vi "FTW-Test-Actor-Core_Process.vi"(0 "FTW Actor Instance Configuration":string="{\n  \"Identity\": \"ActorName\",\n  \"InboxAddress\": \"inproc://*\",\n  \"LoggerAddress\": \"\",\n  \"My Data\": false,\n  \"Publisher URI\": \"inproc://*\",\n  \"Subscriber URIs\": \"\",\n  \"Refresh Period\": 2\n}", 11 "ErrorIn":errorcluster) -> (15 "Error":errorcluster)   [LabVIEW 2015, in "FTW-Test-Actor-Core.lvclass"]
uses:
  FTW-Test-Actor-Core.lvclass
  source/actor/Message/Base/FTW-Message.lvclass
  FTW-Test-Actor-Core.lvclass/FTW-Test-Actor-Core.ctl
  source/actor/Instance/FTW-ActorInstance.lvclass/FTW-ActorInstance.ctl
  source/actor/JobSequencer/FTW-SEQ-Current.vi
  source/actor/Connector/FTW-ActorConnector.lvclass
  source/actor/Instance/FTW-ActorInstance.lvclass
  source/actor/Message/Request/FTW-Message-IncomingRequest.lvclass
  source/actor/Publisher/FTW-Publisher.lvclass
  source/actor/Subscriber/FTW-Subscriber.lvclass
panel:
  # "#TODO\nhide controls for a GUI"
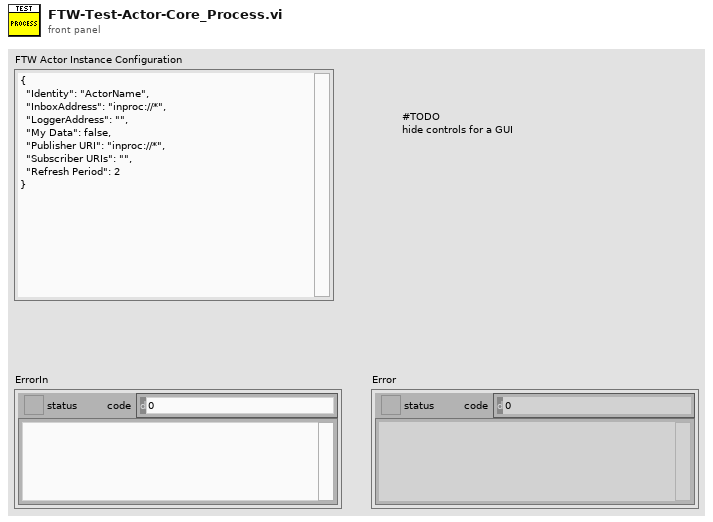
[diagram p1: front panel]
types:
  T1 = cluster{"Incoming Requests":refnum<event-registration>, "Local Messages":refnum<event-registration>, "Subscription":refnum<event-registration>}
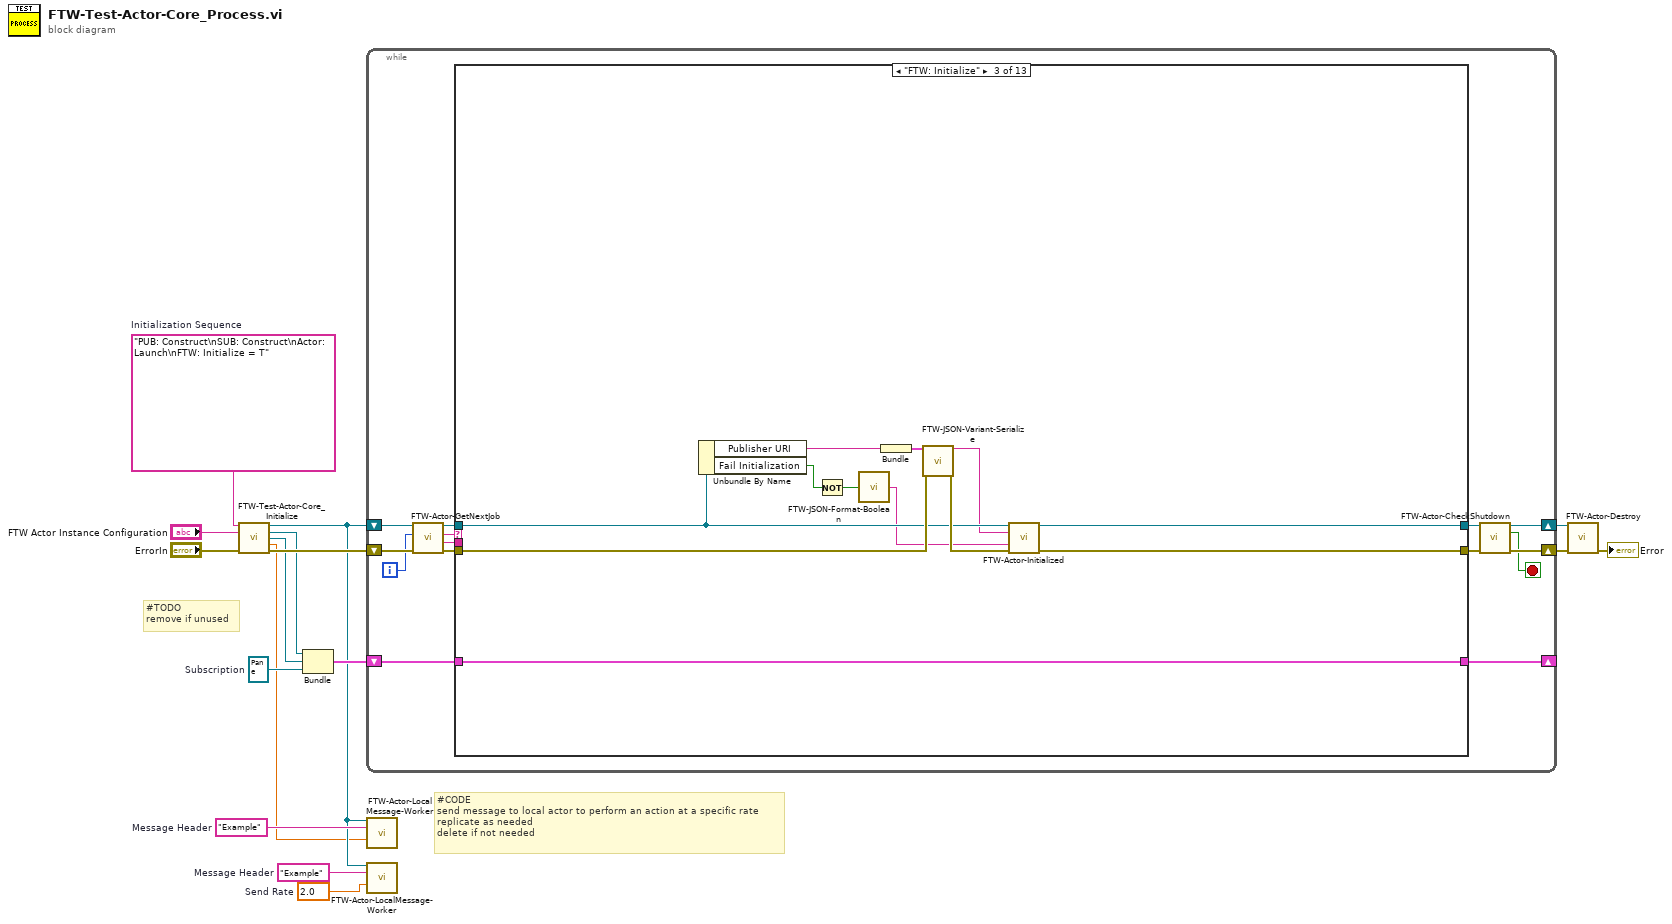
[diagram p0: block diagram]
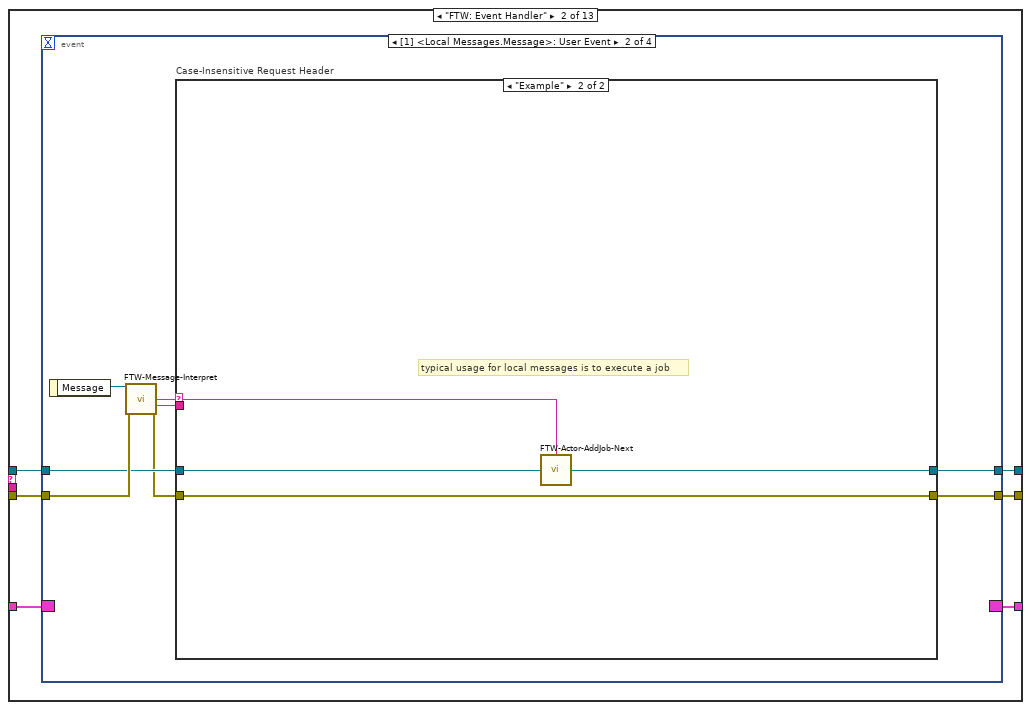
[diagram p3: hidden frame]
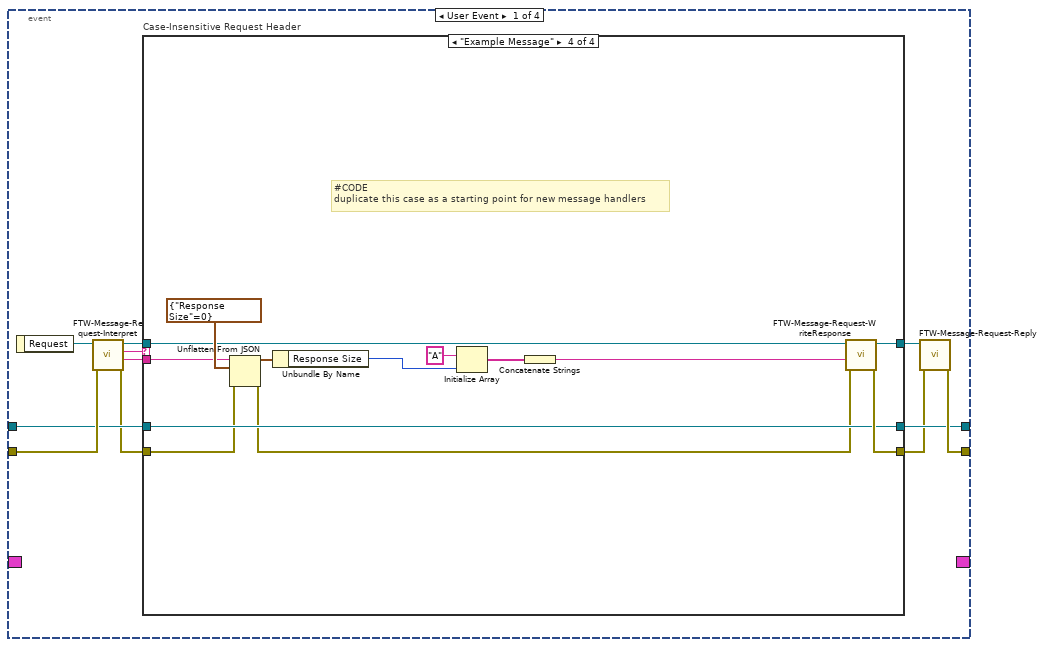
[diagram p4: hidden frame]
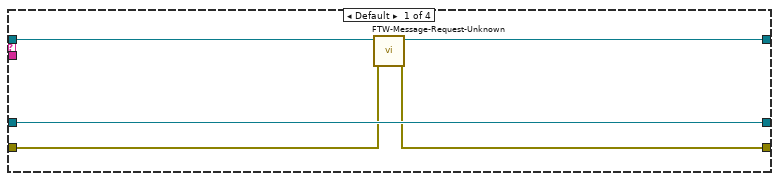
[diagram p5: hidden frame]
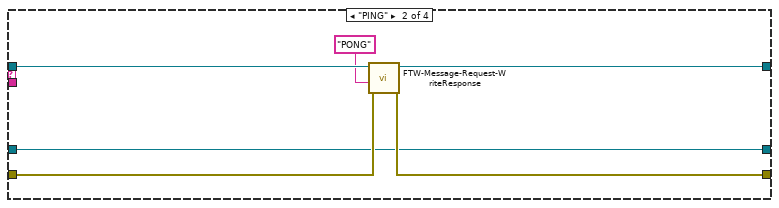
[diagram p6: hidden frame]
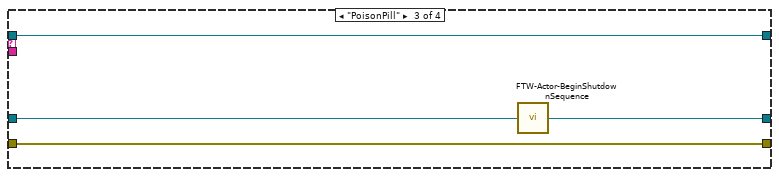
[diagram p7: hidden frame]
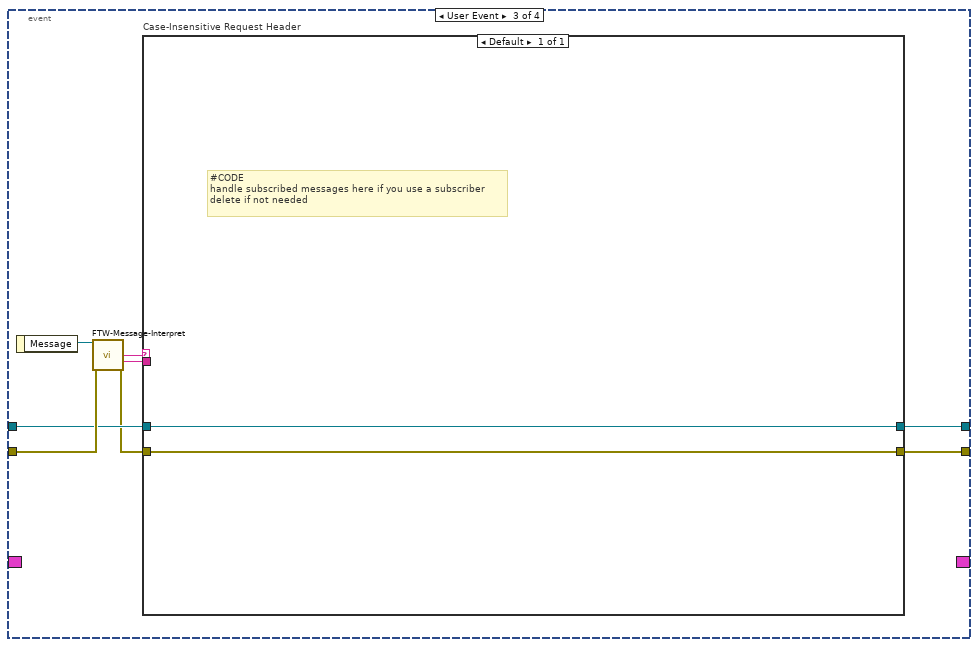
[diagram p9: hidden frame]
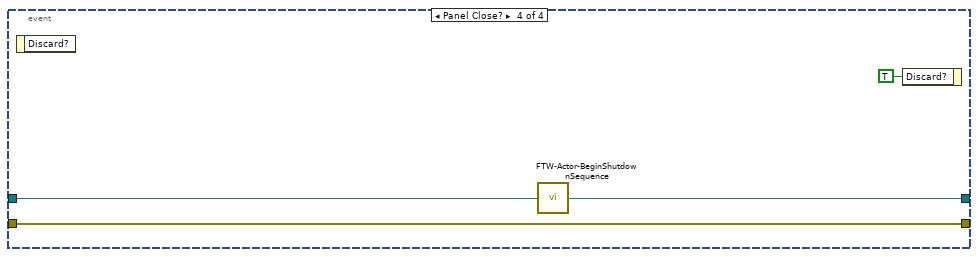
[diagram p10: hidden frame]
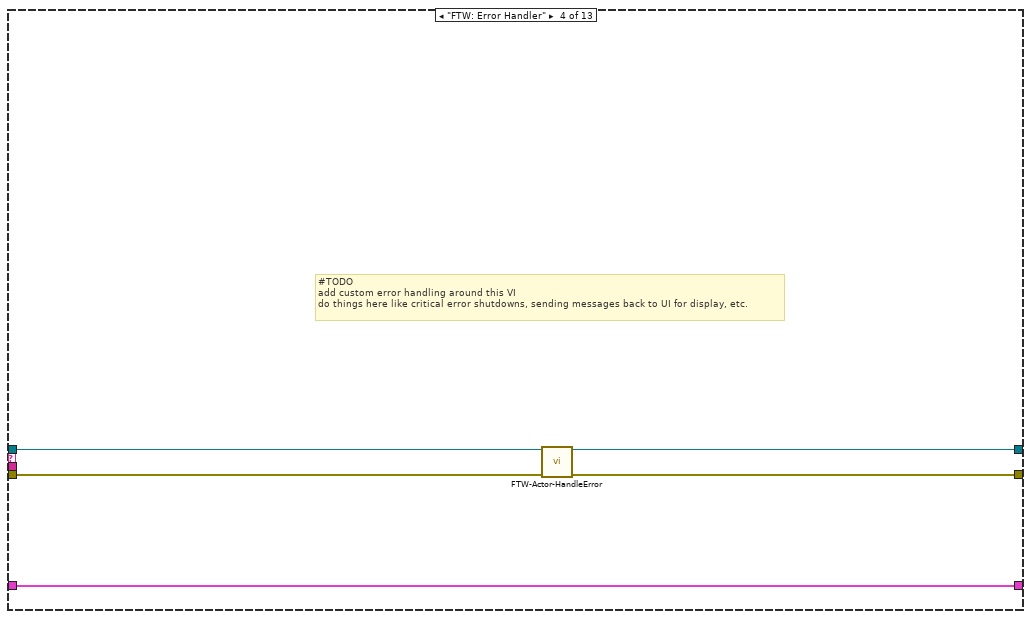
[diagram p11: hidden frame]
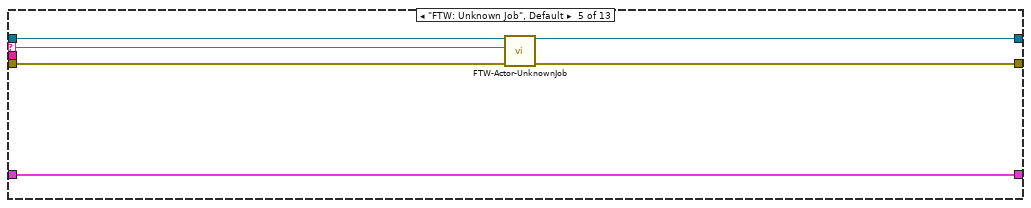
[diagram p12: hidden frame]
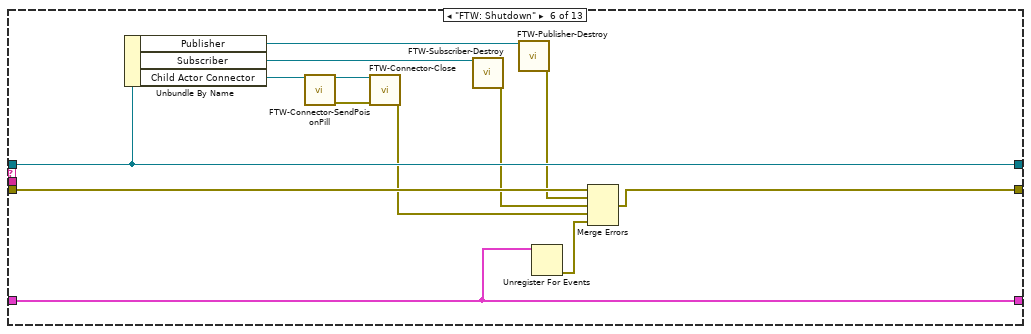
[diagram p13: hidden frame]
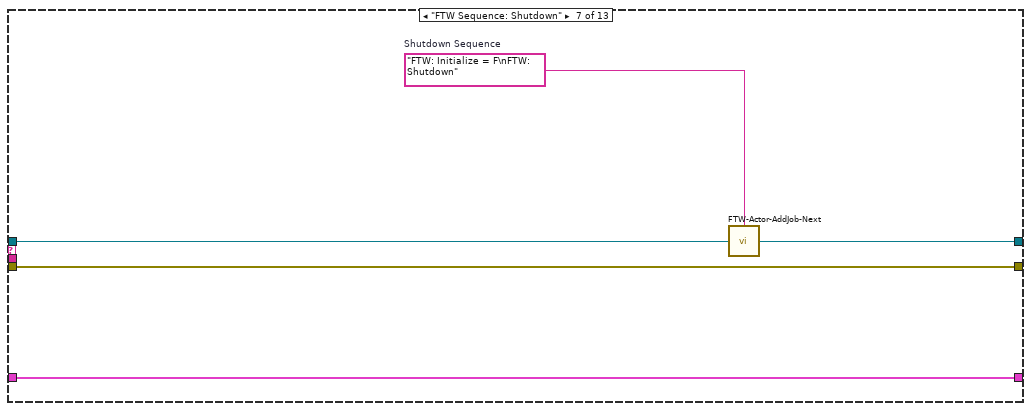
[diagram p14: hidden frame]
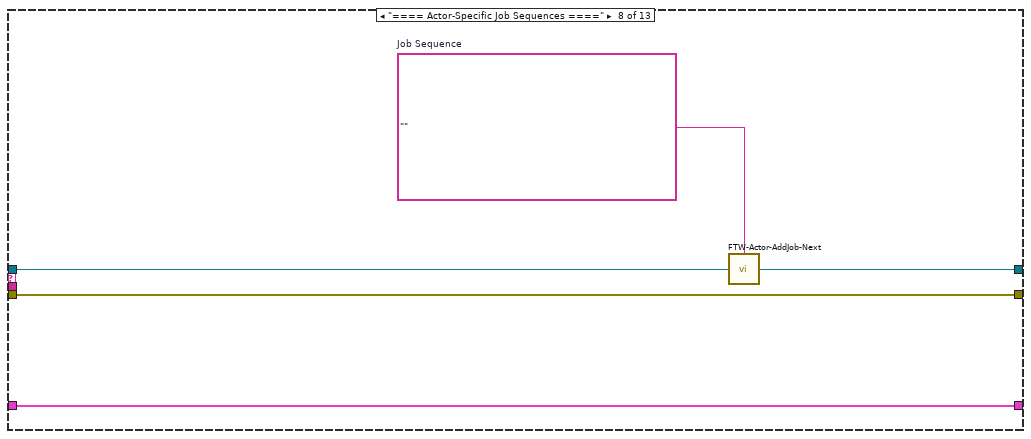
[diagram p15: hidden frame]
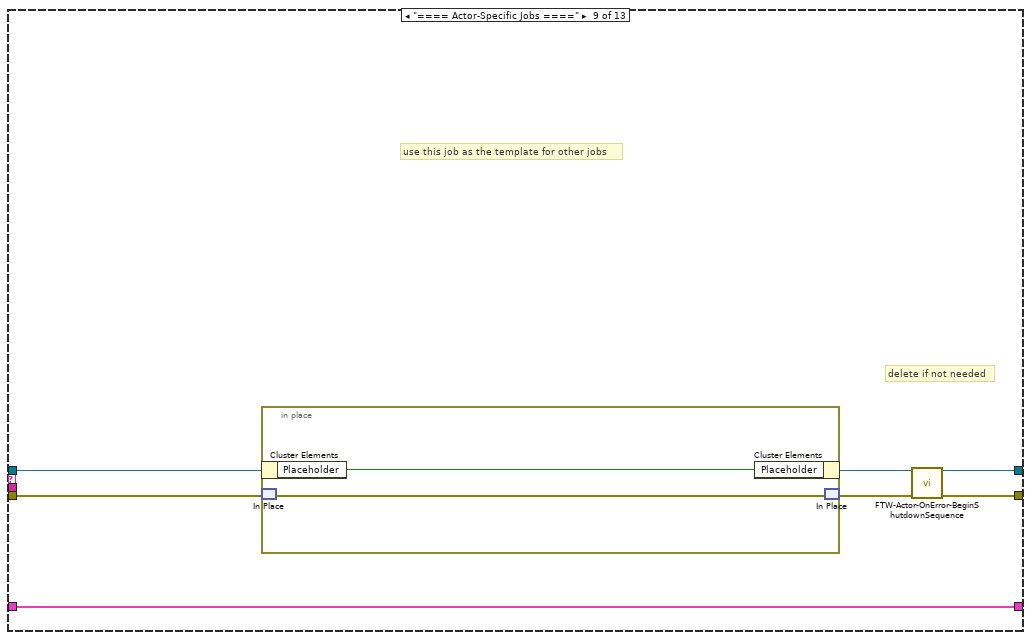
[diagram p16: hidden frame]
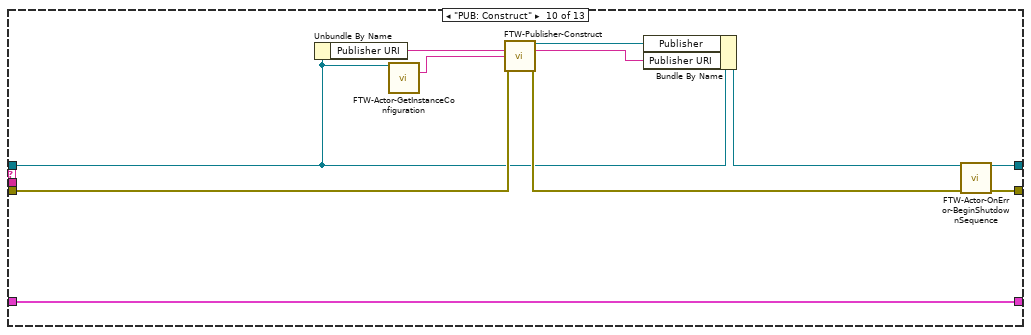
[diagram p17: hidden frame]
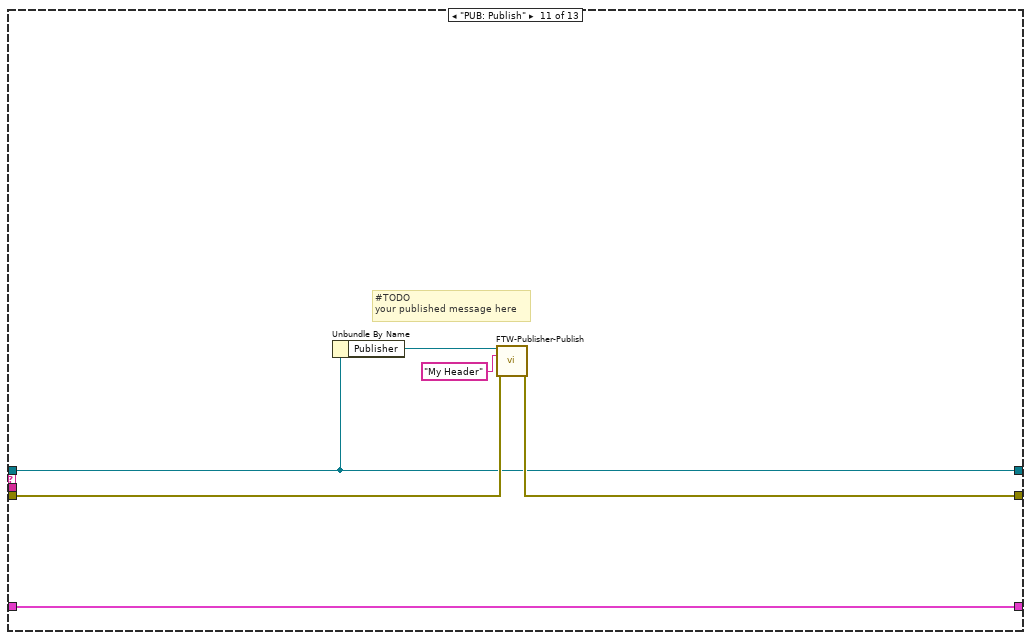
[diagram p18: hidden frame]
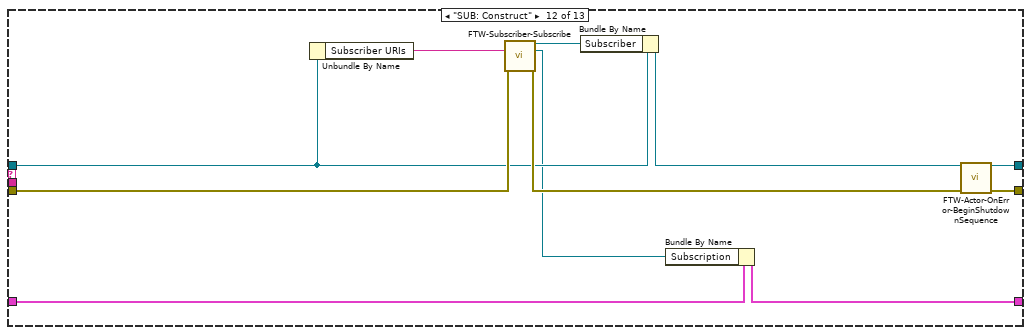
[diagram p19: hidden frame]
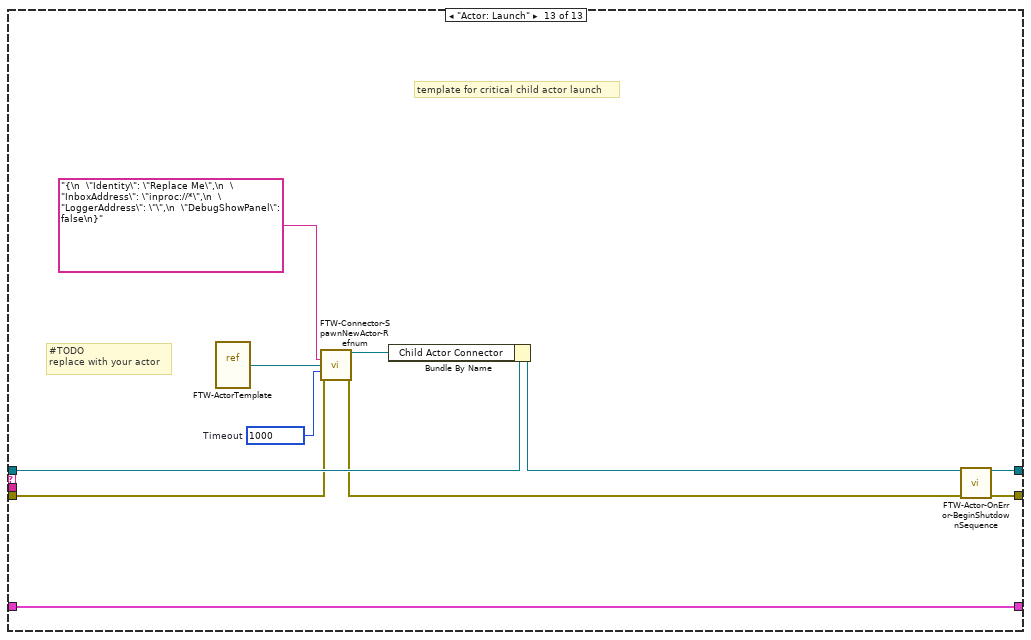
[diagram p20: hidden frame]
diagram:
  w4 = 2.0  # Send Rate
  w3 = "Example"  # Message Header
  w5 = "Example"  # Message Header
  w6 = refnum<event-registration> refnum  # Subscription
  w12 = "PUB: Construct\nSUB: Construct\nActor: Launch\nFTW: Initialize = T"  # Initialization Sequence
  # "#CODE\nsend message to local actor to perform an action at a specific rate\nreplicate as needed\ndelete if not needed"
  # "#TODO\nremove if unused"
  n1 = call "FTW-Test-Actor-Core_Initialize.vi"("Initialization Sequence"=w12, "FTW Actor Instance Configuration"="FTW Actor Instance Configuration", "error in (no error)"="ErrorIn") -> ("Actor Template-Core out"=w2:refnum<class "FTW-Test-Actor-Core.lvclass">, "Incoming Requests"=w8:refnum<event-registration>, "Local Messages"=w7:refnum<event-registration>, "Refresh Period"=w1:dbl, "error out"=w13:errorcluster)  [unwired: 8 in]
  n2 = Bundle("Incoming Requests"=w8, "Local Messages"=w7, "Subscription"=w6) -> (w10:T1)  [unwired: 1 in]
  n3 = while {
    shift-right: [w20] -> w15
    shift-left: w13 -> [w27]
    shift-right: [w17] -> _
    shift-left: w10 -> [w30]
    shift-right: [w22] -> w16
    shift-left: w2 -> [w29]
    i -> [w18]
    stop <- w19 stop-if-true
    n4 = call "FTW-Actor-GetNextJob.vi"("error in"=w27, "Jobs Performed"=w18, "FTW Actor Instance"=w29) -> ("error out"=w26:errorcluster, "Job Data"=w24:string, "Job Name"=w25:string, "FTW Actor Instance out"=w28:refnum<class "FTW-Test-Actor-Core.lvclass">)  [unwired: 5 in]
    n5 = case shown="\"FTW: Initialize\"" w25 {
      selector: w25 -> [_ _ _ _ w124 _ _ _ _ _ _ _ _]
      tunnel: [w32 w39 w114 w119 w127 w141 w146 w151 w155 w168 w176 w185 w199] -> w21
      tunnel: w26 -> [w32 w38 w118 w121 w128 w142 w146 w151 w158 w170 w177 w187 w193]
      tunnel: w30 -> [w33 w34 w116 w123 w129 w139 w147 w152 w159 w172 w178 w189 w200]
      tunnel: [w33 w37 w116 w123 w129 w139 w147 w152 w159 w172 w178 w180 w200] -> w17
      tunnel: w24 -> [_ _ _ _ _ _ _ _ _ _ _ _ _]
      tunnel: [w31 w36 w115 w120 w125 w138 w144 w149 w153 w166 w175 w183 w198] -> w23
      tunnel: w28 -> [w31 w35 w113 w122 w126 w138 w145 w150 w156 w163 w175 w181 w197]
      frame "==== Featherweight Framework Jobs ====" {
      }
      frame "FTW: Event Handler" {
        n6 = event shown="[1] <Local Messages.Message>: User Event" {
          selector: w34 -> [_ _ _ _]
          dyn-events: [_ _ _ _] -> w37
          timeout: _ -> [_ _ _ _]
          tunnel: [w49 w81 w95 w105] -> w39
          tunnel: w38 -> [w48 w85 w99 w105]
          tunnel: [w43 w82 w96 w103] -> w36
          tunnel: w35 -> [w47 w84 w98 w104]
          event User Event {
            n7 = event-data() -> ("Request"=w50:refnum<class "FTW-Message-IncomingRequest.lvclass">)  [unwired: 1 in]
            n8 = call "FTW-Message-Request-Interpret.vi"("error in"=w48, "FTW Incoming Request"=w50) -> ("error out"=w46:errorcluster, "Request Body"=w40:string, "Request Header"=w44:string, "FTW Incoming Request out"=w45:refnum<class "FTW-Message-IncomingRequest.lvclass">)  [unwired: 6 in]
            n9 = case "Case-Insensitive Request Header" shown="\"Example Message\"" w44 {
              tunnel: [w53 w59 w64 w78] -> w42
              tunnel: w46 -> [w54 w60 w64 w67]
              tunnel: [w55 w58 w65 w76] -> w43
              tunnel: w47 -> [w55 w58 w63 w76]
              tunnel: w45 -> [w52 w61 w62 w68]
              tunnel: [w51 w57 w62 w77] -> w41
              tunnel: w40 -> [_ _ _ w66]
              frame Default {
                n10 = call "FTW-Message-Request-Unknown.vi"("error in"=w54, "FTW Incoming Request"=w52) -> ("error out"=w53:errorcluster, "FTW Incoming Request Out"=w51:refnum<class "FTW-Message-IncomingRequest.lvclass">)  [unwired: 8 in]
              }
              frame "PING" {
                n11 = call "FTW-Message-Request-WriteResponse.vi"("error in"=w60, "Response Body"="PONG" ("Response Header"), "FTW Incoming Request"=w61) -> ("error out"=w59:errorcluster, "FTW Incoming Request out"=w57:refnum<class "FTW-Message-IncomingRequest.lvclass">)  [unwired: 7 in]
              }
              frame "PoisonPill" {
                n12 = call "FTW-Actor-BeginShutdownSequence.vi"("FTW Actor Instance"=w63) -> ("FTW Actor Instance out"=w65:refnum<class "FTW-Test-Actor-Core.lvclass">)  [unwired: 3 in]
              }
              frame "Example Message" {
                # "#CODE\nduplicate this case as a starting point for new message handlers"
                n13 = Unflatten From JSON(JSON string=w66, type and defaults=cluster{"Response Size":i32} {"Response Size"=0}, error in (no error)=w67) -> (value=w73:cluster{"Response Size":i32}, error out=w75:errorcluster)  [unwired: 4 in]
                n14 = Unbundle By Name(w73) -> ("Response Size"=w72:i32)
                n15 = Initialize Array("A", w72) -> (w70:string[])
                n16 = Concatenate Strings(w70) -> (w69:string)
                n17 = call "FTW-Message-Request-WriteResponse.vi"("error in"=w75, "Response Body"=w69, "FTW Incoming Request"=w68) -> ("error out"=w78:errorcluster, "FTW Incoming Request out"=w77:refnum<class "FTW-Message-IncomingRequest.lvclass">)  [unwired: 7 in]
              }
            }
            n18 = call "FTW-Message-Request-Reply.vi"("FTW: Reply Error"=w42, "FTW Incoming Request"=w41) -> ("error out"=w49:errorcluster)  [unwired: 8 in, 1 out]
          }
          event User Event {
            n19 = event-data() -> ("Message"=w86:refnum<class "FTW-Message.lvclass">)  [unwired: 1 in]
            n20 = call-dynamic "FTW-Message-Interpret.vi"("FTW Message"=w86, "error in"=w85) -> ("Message Header"=w80:string, "Message Body"=w79:string, "error out"=w83:errorcluster)  [unwired: 9 in, 2 out]
            n21 = case "Case-Insensitive Request Header" shown="\"Example\"" w80 {
              selector: w80 -> [_ w89]
              tunnel: [w87 w91] -> w81
              tunnel: w83 -> [w87 w91]
              tunnel: [w88 w90] -> w82
              tunnel: w84 -> [w88 w92]
              tunnel: w79 -> [_ _]
              frame Default {
                # "#CODE\nhandle local messages here\ndelete if not needed"
              }
              frame "Example" {
                # "typical usage for local messages is to execute a job"
                n22 = call "FTW-Actor-AddJob-Next.vi"("Add Next in Job Queue"=w89, "FTW Actor Instance"=w92) -> ("FTW Actor Instance out"=w90:refnum<class "FTW-Test-Actor-Core.lvclass">)  [unwired: 2 in]
              }
            }
          }
          event User Event {
            n23 = event-data() -> ("Message"=w100:refnum<class "FTW-Message.lvclass">)  [unwired: 1 in]
            n24 = call-dynamic "FTW-Message-Interpret.vi"("FTW Message"=w100, "error in"=w99) -> ("Message Header"=w94:string, "Message Body"=w93:string, "error out"=w97:errorcluster)  [unwired: 9 in, 2 out]
            n25 = case "Case-Insensitive Request Header" shown="Default" w94 {
              tunnel: [w101] -> w95
              tunnel: w97 -> [w101]
              tunnel: [w102] -> w96
              tunnel: w98 -> [w102]
              tunnel: w93 -> [_]
              frame Default {
                # "#CODE\nhandle subscribed messages here if you use a subscriber\ndelete if not needed"
              }
            }
          }
          event Panel Close? {
            n26 = event-data() -> ()  [unwired: 1 in, 1 out]
            n27 = call "FTW-Actor-BeginShutdownSequence.vi"("FTW Actor Instance"=w104) -> ("FTW Actor Instance out"=w103:refnum<class "FTW-Test-Actor-Core.lvclass">)  [unwired: 3 in]
            n28 = event-data("Discard?"=TRUE) -> ()  [unwired: 1 in, 1 out]
          }
        }
      }
      frame "FTW: Initialize" {
        n29 = Unbundle By Name(w113) -> ("Publisher URI"=w112:string, "Fail Initialization"=w109:bool)
        n30 = Not(x=w109) -> (.not. x?=w107:bool)
        n31 = call "FTW-JSON-Format-Boolean.vi"("LabVIEW Boolean"=w107) -> ("JSON Boolean"=w108:string)
        n32 = Bundle("Publisher URI"=w112) -> (w111:cluster{"Publisher URI":string})  [unwired: 1 in]
        n33 = call "FTW-JSON-Variant-Serialize.vi"("Variant"=w111, "error in"=w118) -> ("JSON String"=w110:string, "error out"=w117:errorcluster)  [unwired: 12 in]
        n34 = call-dynamic "FTW-Actor-Initialized.vi"("FTW Actor Instance"=w113, "Initialized Response"=w110, "Positive Init?"=w108, "error in"=w117) -> ("FTW Actor Instance out"=w115:refnum<class "FTW-Test-Actor-Core.lvclass">, "error out"=w114:errorcluster)  [unwired: 10 in]
      }
      frame "FTW: Error Handler" {
        # "#TODO\nadd custom error handling around this VI\ndo things here like critical error shutdowns, sending messages back to UI for display, etc."
        n35 = call-dynamic "FTW-Actor-HandleError.vi"("FTW Actor Instance"=w122, "error in"=w121) -> ("FTW Actor Instance out"=w120:refnum<class "FTW-Test-Actor-Core.lvclass">, "error out"=w119:errorcluster)  [unwired: 10 in, 2 out]
      }
      frame "FTW: Unknown Job", Default {
        n36 = call-dynamic "FTW-Actor-UnknownJob.vi"("FTW Actor Instance"=w126, "Unknown Job"=w124, "error in"=w128) -> ("FTW Actor Instance out"=w125:refnum<class "FTW-Test-Actor-Core.lvclass">, "error out"=w127:errorcluster)  [unwired: 11 in]
      }
      frame "FTW: Shutdown" {
        n37 = Unbundle By Name(w138) -> ("Publisher"=w137:refnum<class "FTW-Publisher.lvclass">, "Subscriber"=w135:refnum<class "FTW-Subscriber.lvclass">, "Child Actor Connector"=w133:refnum<class "FTW-ActorConnector.lvclass">)
        n38 = call-dynamic "FTW-Connector-SendPoisonPill.vi"("FTW Actor Connector"=w133) -> ("FTW Actor Connector out"=w132:refnum<class "FTW-ActorConnector.lvclass">, "error out"=w131:errorcluster)  [unwired: 9 in, 4 out]
        n39 = call-dynamic "FTW-Connector-Close.vi"("FTW Actor Connector"=w132, "error in"=w131) -> ("error out"=w130:errorcluster)  [unwired: 13 in]
        n40 = call "FTW-Subscriber-Destroy.vi"("FTW-Subscription In"=w135) -> ("error out"=w134:errorcluster)  [unwired: 14 in]
        n41 = call "FTW-Publisher-Destroy.vi"("FTW-Publisher In"=w137) -> ("error out"=w136:errorcluster)  [unwired: 14 in]
        n42 = Unregister For Events(event registration refnum=w139) -> (error out=w140:errorcluster)  [unwired: 1 in]
        n43 = Merge Errors(w142, w136, w134, w130, w140) -> (w141:errorcluster)
      }
      frame "FTW Sequence: Shutdown" {
        w143 = "FTW: Initialize = F\nFTW: Shutdown"  # Shutdown Sequence
        n44 = call "FTW-Actor-AddJob-Next.vi"("Add Next in Job Queue"=w143, "FTW Actor Instance"=w145) -> ("FTW Actor Instance out"=w144:refnum<class "FTW-Test-Actor-Core.lvclass">)  [unwired: 2 in]
      }
      frame "==== Actor-Specific Job Sequences ====" {
        w148 = ""  # Job Sequence
        n45 = call "FTW-Actor-AddJob-Next.vi"("Add Next in Job Queue"=w148, "FTW Actor Instance"=w150) -> ("FTW Actor Instance out"=w149:refnum<class "FTW-Test-Actor-Core.lvclass">)  [unwired: 2 in]
      }
      frame "==== Actor-Specific Jobs ====" {
        # "delete if not needed"
        # "use this job as the template for other jobs"
        n46 = in-place {
          n47 = in-place-cluster #1(w156) -> ("Placeholder"=w160:bool)
          n48 = in-place-match #2(w158) -> (w161:errorcluster)
          n49 = in-place-cluster #1("Placeholder"=w160) -> (w154:refnum<class "FTW-Test-Actor-Core.lvclass">)
          n50 = in-place-match #2(w161) -> (w157:errorcluster)
        }
        n51 = call-dynamic "FTW-Actor-OnError-BeginShutdownSequence.vi"("FTW Actor Instance"=w154, "error in"=w157) -> ("FTW Actor Instance out"=w153:refnum<class "FTW-Test-Actor-Core.lvclass">, "error out"=w155:errorcluster)  [unwired: 12 in]
      }
      frame "PUB: Construct" {
        n52 = Unbundle By Name(w163) -> ("Publisher URI"=w164:string)
        n53 = call "FTW-Actor-GetInstanceConfiguration.vi"("FTW Actor Instance"=w163) -> ("Identity"=w162:string)  [unwired: 12 in, 2 out]
        n54 = call "FTW-Publisher-Construct.vi"("Address"=w164, "Identity"=w162, "error in"=w170) -> ("FTW-Publisher Out"=w171:refnum<class "FTW-Publisher.lvclass">, "Actual Address"=w165:string, "error out"=w169:errorcluster)  [unwired: 10 in]
        n55 = Bundle By Name(cluster=w163, "Publisher"=w171, "Publisher URI"=w165) -> (w167:refnum<class "FTW-Test-Actor-Core.lvclass">)
        n56 = call-dynamic "FTW-Actor-OnError-BeginShutdownSequence.vi"("FTW Actor Instance"=w167, "error in"=w169) -> ("FTW Actor Instance out"=w166:refnum<class "FTW-Test-Actor-Core.lvclass">, "error out"=w168:errorcluster)  [unwired: 12 in]
      }
      frame "PUB: Publish" {
        # "#TODO\nyour published message here"
        n57 = Unbundle By Name(w175) -> ("Publisher"=w174:refnum<class "FTW-Publisher.lvclass">)
        n58 = call "FTW-Publisher-Publish.vi"("FTW-Publisher In"=w174, "Header"="My Header", "error in"=w177) -> ("error out"=w176:errorcluster)  [unwired: 11 in, 1 out]
      }
      frame "SUB: Construct" {
        n59 = Unbundle By Name(w181) -> ("Subscriber URIs"=w182:string)
        n60 = call "FTW-Subscriber-Subscribe.vi"("Addresses"=w182, "error in"=w187) -> ("FTW-Subscription Out"=w188:refnum<class "FTW-Subscriber.lvclass">, "Subscriber Registration"=w179:refnum<event-registration>, "error out"=w186:errorcluster)  [unwired: 11 in]
        n61 = Bundle By Name(cluster=w181, "Subscriber"=w188) -> (w184:refnum<class "FTW-Test-Actor-Core.lvclass">)
        n62 = Bundle By Name(cluster=w189, "Subscription"=w179) -> (w180:T1)
        n63 = call-dynamic "FTW-Actor-OnError-BeginShutdownSequence.vi"("FTW Actor Instance"=w184, "error in"=w186) -> ("FTW Actor Instance out"=w183:refnum<class "FTW-Test-Actor-Core.lvclass">, "error out"=w185:errorcluster)  [unwired: 12 in]
      }
      frame "Actor: Launch" {
        w196 = 1000  # Timeout
        # "#TODO\nreplace with your actor"
        # "template for critical child actor launch"
        n64 = vi-ref "FTW-ActorTemplate.vi"() -> (w195:refnum<vi>)
        n65 = call "FTW-Connector-SpawnNewActor-Refnum.vi"("Configuration"="{\n  \"Identity\": \"Replace Me\",\n  \"InboxAddress\": \"inproc://*\",\n  \"LoggerAddress\": \"\",\n  \"DebugShowPanel\": false\n}", "Actor VI Refnum"=w195, "Timeout"=w196, "error in"=w193) -> ("FTW Actor Connector"=w190:refnum<class "FTW-ActorConnector.lvclass">, "error out"=w192:errorcluster)  [unwired: 8 in, 2 out]
        n66 = Bundle By Name(cluster=w197, "Child Actor Connector"=w190) -> (w191:refnum<class "FTW-Test-Actor-Core.lvclass">)
        n67 = call-dynamic "FTW-Actor-OnError-BeginShutdownSequence.vi"("FTW Actor Instance"=w191, "error in"=w192) -> ("FTW Actor Instance out"=w198:refnum<class "FTW-Test-Actor-Core.lvclass">, "error out"=w199:errorcluster)  [unwired: 12 in]
      }
    }
    n68 = call "FTW-Actor-CheckShutdown.vi"("FTW Actor Instance"=w23, "error in"=w21) -> ("FTW Actor Instance out"=w22:refnum<class "FTW-Test-Actor-Core.lvclass">, "Shutdown?"=w19:bool, "error out"=w20:errorcluster)  [unwired: 11 in]
  }
  n69 = call-dynamic "FTW-Actor-LocalMessage-Worker.vi"("FTW-ActorInstance In"=w2, "Message Header"=w5, "Send Rate"=w1) -> ()  [unwired: 13 in]
  n70 = call-dynamic "FTW-Actor-LocalMessage-Worker.vi"("FTW-ActorInstance In"=w2, "Message Header"=w3, "Send Rate"=w4) -> ()  [unwired: 13 in]
  n71 = call-dynamic "FTW-Actor-Destroy.vi"("FTW Actor Instance"=w16, "error in"=w15) -> ("error out"=→"Error":errorcluster)  [unwired: 13 in]
